vi "AlliGator Find Optimal Phasor Calibration (no Starting Calibration).vi"(6 "Use z1 as calibration (T)":bool=TRUE, 8 "Error In":errorcluster, 9 "Phasor Frequency":dbl[unit]) -> (0 "Error Out":errorcluster, 1 "tau 2":dbl[unit], 2 "tau 1":dbl[unit], 3 "Calibration Phasor (g, s)":T1, 4 "Message":string)   [LabVIEW 2021, in "AlliGator Phasor Calibration.lvlib"]
doc: "Find optimal <B.Calibration Phasor</B> for the two existing phasor references."
uses:
  AlliGator Phasor Calibration.lvlib
  Phasor/Phasor (g, s).ctl
  <vilib>/Utility/error.llb/DialogType.ctl
  AlliGator ucno_objective function phasor calibration.vi
  <vilib>/gmath/NumericalOptimization/Quasi Newton.vi
  Phasor/Phasor.lvlib
  <vilib>/gmath/NI_Gmath.lvlib
  AlliGator Phasor Ratio.lvlib
  Variant/Variant.lvlib
panel:
  out "number of function evaluations":i32
  out "f(minimum)":dbl
  # "see the AlliGator License on the block diagram (Ctrl+E or Window:Show Block Diagram)"
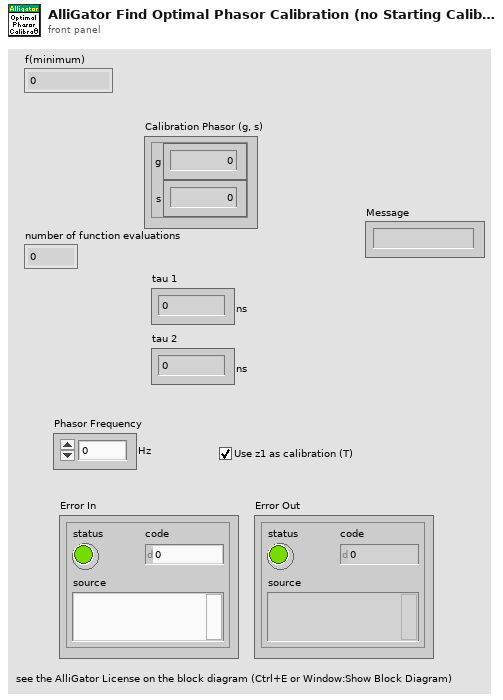
[diagram p1: front panel]
types:
  T1 = typedef "Phasor.lvlib/Phasor (g, s).ctl" = cluster{"g":dbl, "s":dbl}
  T2 = typedef "Phasor.lvlib/Phasor (m, phi).ctl" = cluster{"m":dbl, "phi":dbl}
  T3 = typedef "DialogType.ctl" = u16
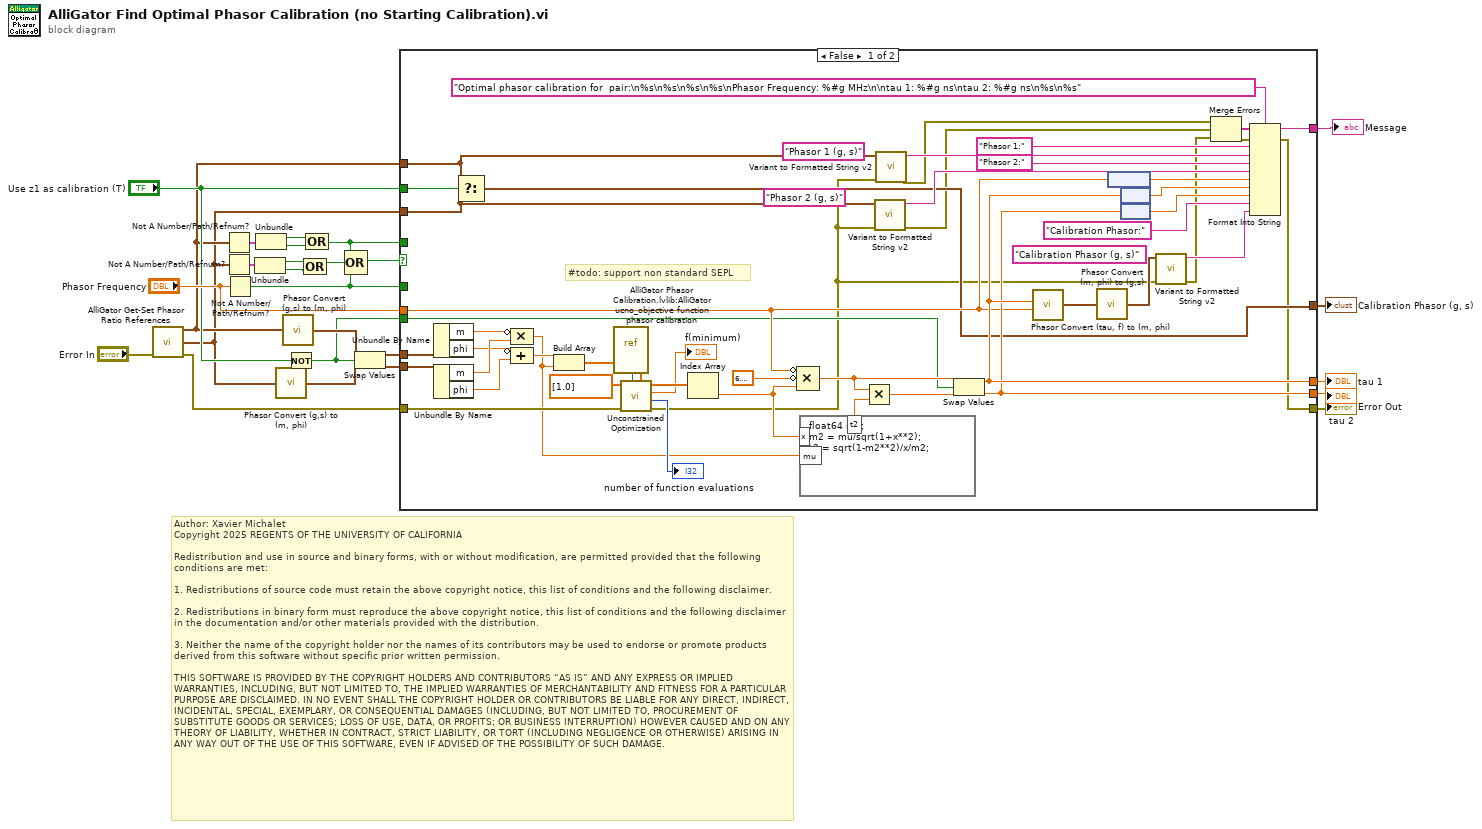
[diagram p0: block diagram]
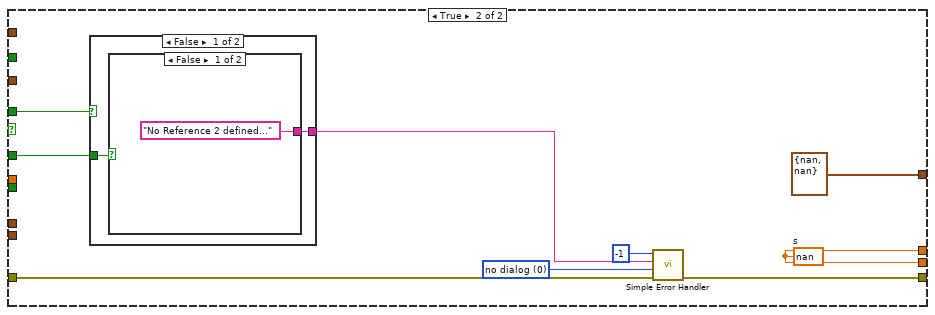
[diagram p2: hidden frame]
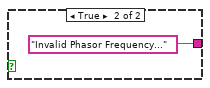
[diagram p3: hidden frame]
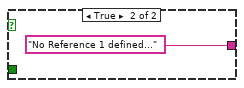
[diagram p4: hidden frame]
diagram:
  # "Author: Xavier Michalet\nCopyright 2025 REGENTS OF THE UNIVERSITY OF CALIFORNIA\n\nRedistribution and use in source and binary forms, with or without modification, are permitted provided that the following conditions are met:\n\n1. Redistributions of source code must retain the above copyright notice, this list of conditions and the following disclaimer.\n\n2. Redistributions in binary form must reproduce the above copyright notice, this list of conditions and the following disclaimer in the documentation and/or other materials provided with the distribution.\n\n3. Neither the name of the copyright holder nor the names of its contributors may be used to endorse or promote products derived from this software without specific prior written permission.\n\nTHIS SOFTWARE IS PROVIDED BY THE COPYRIGHT HOLDERS AND CONTRIBUTORS “AS IS” AND ANY EXPRESS OR IMPLIED WARRANTIES, INCLUDING, BUT NOT LIMITED TO, THE IMPLIED WARRANTIES OF MERCHANTABILITY AND FITNESS FOR A PARTICULAR PURPOSE ARE DISCLAIMED. IN NO EVENT SHALL THE COPYRIGHT HOLDER OR CONTRIBUTORS BE LIABLE FOR ANY DIRECT, INDIRECT, INCIDENTAL, SPECIAL, EXEMPLARY, OR CONSEQUENTIAL DAMAGES (INCLUDING, BUT NOT LIMITED TO, PROCUREMENT OF SUBSTITUTE GOODS OR SERVICES; LOSS OF USE, DATA, OR PROFITS; OR BUSINESS INTERRUPTION) HOWEVER CAUSED AND ON ANY THEORY OF LIABILITY, WHETHER IN CONTRACT, STRICT LIABILITY, OR TORT (INCLUDING NEGLIGENCE OR OTHERWISE) ARISING IN ANY WAY OUT OF THE USE OF THIS SOFTWARE, EVEN IF ADVISED OF THE POSSIBILITY OF SUCH DAMAGE."
  n1 = call "AlliGator Get-Set Phasor Ratio References.vi"("error in (no error)"="Error In") -> ("Reference Phasor 1"=w5:T1, "Reference Phasor 2"=w4:T1, "error out"=w2:errorcluster)  [unwired: 7 in, 5 out]
  n2 = Not A Number/Path/Refnum?(number/path/refnum=w5) -> (NaN/Path/Refnum?=w16:cluster{"g":bool, "s":bool})
  n3 = Not A Number/Path/Refnum?(number/path/refnum=w4) -> (NaN/Path/Refnum?=w15:cluster{"g":bool, "s":bool})
  n4 = Not A Number/Path/Refnum?(number/path/refnum="Phasor Frequency") -> (NaN/Path/Refnum?=w7:bool)
  n5 = Unbundle(w15) -> ("g"=w12:bool, "s"=w11:bool)
  n6 = Unbundle(w16) -> ("g"=w14:bool, "s"=w13:bool)
  n7 = call "Phasor Convert (g,s) to (m, phi).vi"("Phasor (g, s)"=w4) -> ("Phasor (m, phi)"=w25:T2)  [unwired: 8 in]
  n8 = call "Phasor Convert (g,s) to (m, phi).vi"("Phasor (g, s)"=w5) -> ("Phasor (m, phi)"=w26:T2)  [unwired: 8 in]
  n9 = Not(x="Use z1 as calibration (T)") -> (.not. x?=w22:bool)
  n10 = Compound Arithmetic op=OR(w12, w11) -> (w10:bool)
  n11 = Compound Arithmetic op=OR(w14, w13) -> (w8:bool)
  n12 = Compound Arithmetic op=OR(w8, w10, w7) -> (w9:bool)
  n13 = Swap Values(12:w26, 13:w22, 14:w25) -> (1:w24:T2, 3:w23:T2)
  n14 = case shown="False" w9 {
    tunnel: w24 -> [w73 _]
    tunnel: w23 -> [w72 _]
    tunnel: w2 -> [w61 w79]
    tunnel: w22 -> [w39 _]
    tunnel: [w28 w79] -> w21
    tunnel: [w50 w81] -> w20
    tunnel: [w48 w81] -> w19
    tunnel: [w36 T1 {"g"=nan, "s"=nan} ("Phasor (g, s)")] -> w18
    tunnel: w5 -> [w38 _]
    tunnel: w4 -> [w37 _]
    tunnel: "Phasor Frequency" -> [w40 _]
    tunnel: w8 -> [_ w77]
    tunnel: w7 -> [_ w74]
    tunnel: "Use z1 as calibration (T)" -> [w35 _]
    tunnel: [w27 _] -> w1
    frame False {
      (unwired) "Calibration Phasor (g, s)" ("Label")
      (unwired) "Phasor 2 (g, s)" ("Label")
      (unwired) "Phasor 1 (g, s)" ("Label")
      # "#todo: support non standard SEPL"
      n15 = Unbundle By Name(w73) -> ("m"=w71:dbl, "phi"=w69:dbl)
      n16 = Unbundle By Name(w72) -> ("m"=w70:dbl, "phi"=w68:dbl)
      n17 = Select(t=w38, s=w35, f=w37) -> (s? t:f=w36:T1)
      n18 = Compound Arithmetic op=MULTIPLY(invert w71, w70) -> (w54:dbl)
      n19 = Compound Arithmetic op=ADD(invert w69, w68) -> (w67:dbl)
      n20 = Build Array(w67, w54) -> (w66:dbl[])
      n21 = vi-ref "AlliGator Phasor Calibration.lvlib:AlliGator ucno_objective function phasor calibration.vi"() -> (w65:refnum<vi>)
      n22 = call-poly <vilib>:"Unconstrained Optimization.vi"("function data"=w66, "objective function"=w65, "error in (no error)"=w61, "start"=dbl[] [1.0]) -> ("error out"=w34:errorcluster, "number of function evaluations"=→"number of function evaluations":i32, "f(minimum)"=→"f(minimum)":dbl, "minimum"=w63:dbl[])  [unwired: 4 in]
      n23 = Index Array(array=w63) -> (element=w58:dbl)  [unwired: 1 in]
      n24 = Compound Arithmetic op=MULTIPLY(invert w40, invert 6.283185307179586, w58) -> (w56:dbl[unit])
      n25 = formula code="float64 m2;\nm2 = mu/sqrt(1+x**2);\nt2 = sqrt(1-m2**2)/x/m2;"("x"=w58, "mu"=w54) -> ("t2"=w57:dbl)
      n26 = Multiply(x=w56, y=w57) -> (x*y=w55:dbl[unit])
      n27 = call "Variant to Formatted String v2.vi"("error in (no error)"=w34, "Anything"=w37) -> ("error out"=w32:errorcluster, "String"=w52:string)  [unwired: 8 in]
      n28 = call "Variant to Formatted String v2.vi"("error in (no error)"=w34, "Anything"=w38) -> ("error out"=w33:errorcluster, "String"=w45:string)  [unwired: 8 in]
      n29 = Swap Values(12:w56, 13:w39, 14:w55) -> (1:w50:dbl[unit], 3:w48:dbl[unit])
      n30 = call "Phasor Convert (tau, f) to (m, phi).vi"("Lifetime"=w50, "Phasor Frequency"=w40) -> ("Phasor (m, phi)"=w29:T2)  [unwired: 5 in]
      n31 = call "Phasor Convert (m, phi) to (g,s).vi"("Phasor (m, phi)"=w29) -> ("Phasor (g, s)"=w46:T1)  [unwired: 8 in]
      n32 = node(w40) -> (w51:dbl)
      n33 = node(w50) -> (w49:dbl)
      n34 = node(w48) -> (w47:dbl)
      n35 = call "Variant to Formatted String v2.vi"("error in (no error)"=w34, "Anything"=w46) -> ("error out"=w30:errorcluster, "String"=w44:string)  [unwired: 8 in]
      n36 = Merge Errors(w33, w32, w30) -> (w31:errorcluster)
      n37 = Format Into String(format string="Optimal phasor calibration for  pair:\n%s\n%s\n%s\n%s\nPhasor Frequency: %#g MHz\n\ntau 1: %#g ns\ntau 2: %#g ns\n%s\n%s", error in=w31, "Phasor 1:" ("Label"), w45, "Phasor 2:" ("Label"), w52, w51, w49, w47, "Calibration Phasor:" ("Label"), w44) -> (resulting string=w27:string, error out=w28:errorcluster)  [unwired: 1 in]
    }
    frame True {
      w75 = T3 0 items=["no dialog", "OK message", "continue or stop message", "OK message + warnings", "continue/stop + warnings"] ("type of dialog (OK msg:1)")
      w81 = dbl[unit] nan  # s
      n38 = case shown="False" w77 {
        tunnel: [w82 "No Reference 1 defined..." ("error source (\" \")")] -> w76
        tunnel: w74 -> [w83 _]
        frame False {
          n39 = case shown="False" w83 {
            tunnel: ["No Reference 2 defined..." ("error source (\" \")") "Invalid Phasor Frequency..." ("error source (\" \")")] -> w82
            frame False {
            }
            frame True {
            }
          }
        }
        frame True {
        }
      }
      n40 = call <vilib>:"Simple Error Handler.vi"("error code (no error:0)"=-1, "error source (\" \")"=w76, "type of dialog (OK msg:1)"=w75) -> ()  [unwired: 2 in, 5 out]
    }
  }
  "Calibration Phasor (g, s)" <- w18
  "tau 1" <- w20
  "tau 2" <- w19
  "Error Out" <- w21
  "Message" <- w1
